vi "ACK 01.vi"(2 "error in (no error)":errorcluster, 3 "RNbits":dbl[](array[numeric])) -> (0 "error out":errorcluster, 1 "ACK array":bool[](array[boolean]))   [LabVIEW 2015]
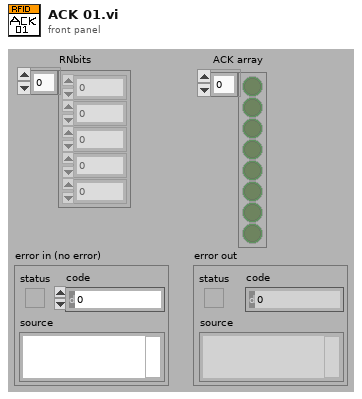
[diagram p1: front panel]
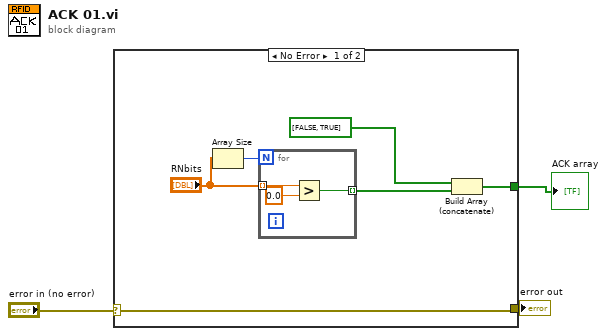
[diagram p0: block diagram]
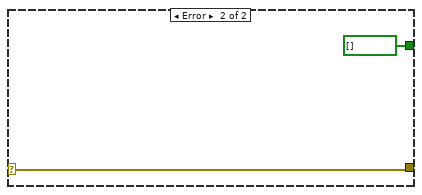
[diagram p2: hidden frame]
diagram:
  n1 = case shown="No Error" "error in (no error)" {
    selector: "error in (no error)" -> [w9 w14]
    tunnel: [w9 w14] -> w2
    tunnel: [w8 bool[] []] -> w1
    frame No Error {
      n2 = Array Size(array="RNbits") -> (size(s)=w6:i32)
      n3 = for {
        N: w6 -> [_]
        tunnel: "RNbits" -> [w12] mode=indexing
        tunnel: [w10] -> w4 mode=indexing
        n4 = Greater?(x=w12, y=0.0) -> (0:w10:bool)
      }
      n5 = Build Array (concatenate)(bool[] [FALSE, TRUE] ("array"), w4) -> (w8:bool[])
    }
    frame Error {
    }
  }
  "error out" <- w2
  "ACK array" <- w1
